vi "Read Choice.vi"(8 "error in (no error)":errorcluster, 11 "_Popup in":refnum<class "Popup.lvclass">) -> (0 "error out":errorcluster, 2 "Choice":bool, 3 "_Popup out":refnum<class "Popup.lvclass">)   [LabVIEW 2021, in "Pop-Up.lvlib" / "Popup.lvclass"]
doc: "This Data Member Access VI will read the choice Boolean from the object.\n\nOutputs: +\n-Choice [Boolean] - the user choice on a two button pop up\n\n<b>Code Developed By:</b> +\nDaniel Coons +\nhttps://github.com/danielcoons/tsc-pop-up"
uses:
  Popup.lvclass
  Popup.lvclass/Popup.ctl
panel:
  # "This VI gets the choice value (boolean) from the Popup Object"
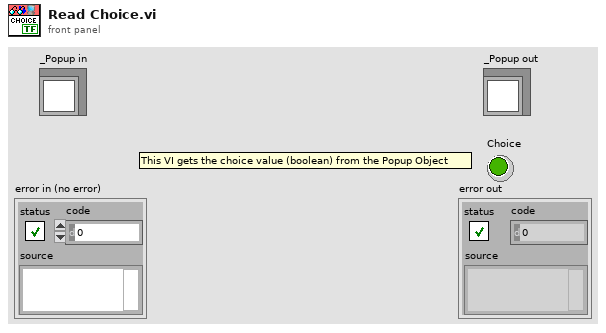
[diagram p1: front panel]
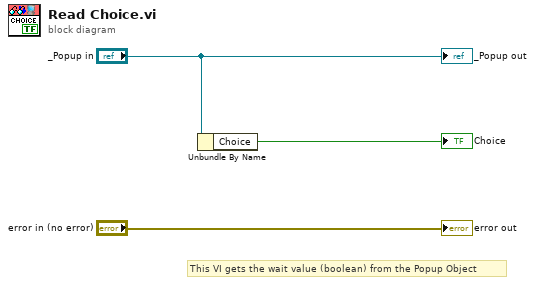
[diagram p0: block diagram]
diagram:
  # "This VI gets the wait value (boolean) from the Popup Object"
  n1 = Unbundle By Name("_Popup in") -> ("Choice"=→"Choice":bool)
  "error out" <- "error in (no error)"
  "_Popup out" <- "_Popup in"
